vi "ValidDragDrop.vi"(8 "error in":errorcluster, 10 "drag over":string, 11 "tree ref in":refnum<vi>) -> (0 "error out":errorcluster, 1 "accepted":bool, 2 "drag":string, 3 "tree ref out":refnum<vi>)   [LabVIEW 2013, in "NISE_CEF_TreeControl.lvlib"]
doc: "This VI is used to see if a drag and drop operation is valid.\nThe drop shoudl be done in a node that accepts that kind of nodes."
uses:
  NISE_CEF_TreeControl.lvlib
  Node/NISE_CEF_Node.lvclass
  Node/SubNodeCluster.ctl
  Node/ReadNodeClass.vi
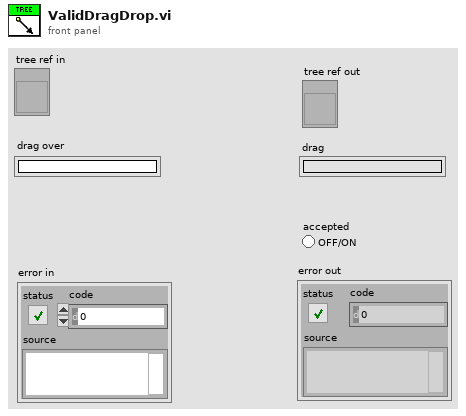
[diagram p1: front panel]
types:
  T1 = typedef "NISE_CEF_Node.lvclass/NodeRef.ctl" = refnum<data-value>
  T2 = typedef "NISE_CEF_Node.lvclass/SubNodeCluster.ctl" = cluster{"subnodes menu name":string[], "subnodes class":string[]}
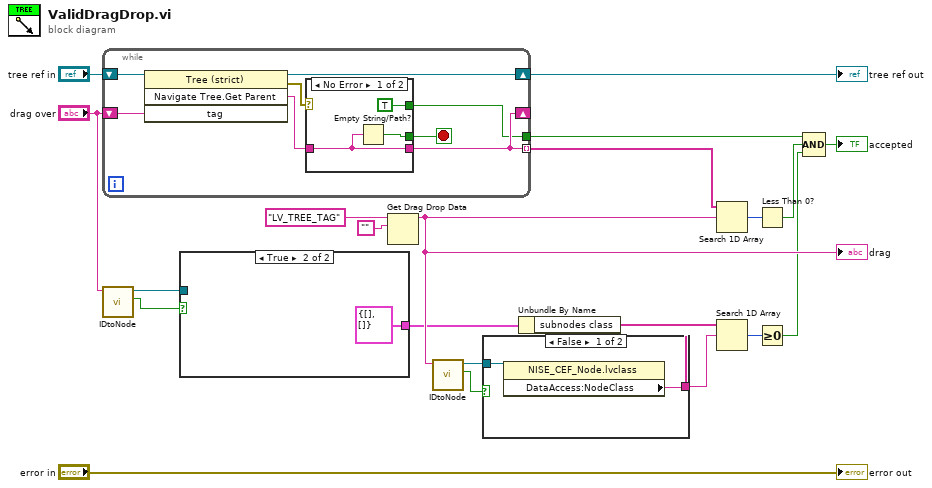
[diagram p0: block diagram]
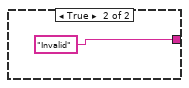
[diagram p2: hidden frame]
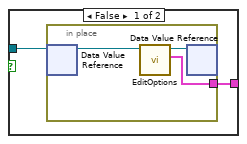
[diagram p3: hidden frame]
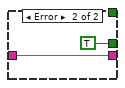
[diagram p4: hidden frame]
diagram:
  n1 = while {
    shift-right: [w24] -> _
    shift-left: "drag over" -> [w28]
    tunnel: [w24] -> w18 mode=indexing
    tunnel: [w23] -> w15
    shift-right: [w22] -> w16
    shift-left: "tree ref in" -> [w29]
    stop <- w27 stop-if-true
    n2 = invoke class="Tree (strict)" method="Navigate Tree.Get Parent"(reference=w29, "tag"=w28) -> (reference out=w22:refnum<vi>, error out=w26:errorcluster, "Navigate Tree:Get Parent"=w25:string)  [unwired: 2 in, 1 out]
    n3 = case shown="No Error" w26 {
      tunnel: [w30 TRUE] -> w27
      tunnel: w25 -> [w31 w33]
      tunnel: [w31 w33] -> w24
      tunnel: [TRUE _] -> w23
      frame No Error {
        n4 = Empty String/Path?(string/path=w31) -> (empty?=w30:bool)
      }
      frame Error {
      }
    }
  }
  "tree ref out" <- w16
  n5 = call "IDtoNode.vi"("ID"="drag over") -> ("invalid Id"=w2:bool, "node ref"=w9:T1)  [unwired: 8 in, 1 out]
  n6 = case shown="True" w2 {
    tunnel: w9 -> [w36 _]
    tunnel: [w35 T2 {"subnodes menu name"=[], "subnodes class"=[]} ("subnodes class")] -> w5
    frame False {
      n7 = in-place {
        in-place-border: [w37] -> w35
        n8 = in-place-dvr #1(w36) -> (w39:refnum<class "NISE_CEF_Node.lvclass">)  [unwired: 1 out]
        n9 = call-dynamic "EditOptions.vi"("node in"=w39) -> ("subnodes class"=w37:T2, "node out"=w38:refnum<class "NISE_CEF_Node.lvclass">)  [unwired: 7 in, 2 out]
        n10 = in-place-dvr #1(w38) -> ()  [unwired: 2 out]
      }
    }
    frame True {
    }
  }
  n11 = Get Drag Drop Data(8:"", 9:"LV_TREE_TAG" ("data name")) -> (3:w12:string)  [unwired: 1 in, 1 out]
  "drag" <- w12
  n12 = call "IDtoNode.vi"("ID"=w12) -> ("invalid Id"=w1:bool, "node ref"=w10:T1)  [unwired: 8 in, 1 out]
  n13 = case shown="False" w1 {
    tunnel: w10 -> [w42 _]
    tunnel: [w41 "Invalid" ("DataAccess:NodeClass")] -> w6
    frame False {
      n14 = property class="NISE_CEF_Node.lvclass"(reference=w42) -> ("DataAccess:NodeClass"=w41:string)  [unwired: 1 in, 2 out]
    }
    frame True {
    }
  }
  n15 = Unbundle By Name(w5) -> ("subnodes class"=w4:string[])
  n16 = Search 1D Array(1D array=w18, element=w12) -> (index of element=w20:i32)  [unwired: 1 in]
  n17 = Search 1D Array(1D array=w4, element=w6) -> (index of element=w8:i32)  [unwired: 1 in]
  n18 = Less Than 0?(x=w20) -> (x < 0?=w14:bool)
  n19 = Greater Or Equal To 0?(x=w8) -> (x >= 0?=w7:bool)
  n20 = Compound Arithmetic op=AND(w15, w14, w7) -> (→"accepted":bool)
  "error out" <- "error in"
